vi "SE Initialization VI.vi"(8 "error in (no error)":errorcluster, 10 "Custom XML":string, 11 "Device Item Ref in":T1 format="%.0x") -> (0 "error out":errorcluster, 3 "Device Item Ref out":T1 format="%.0x")   [LabVIEW 2018, in "Chassis TimeSync System Explorer.lvlib"]
uses:
  Chassis TimeSync System Explorer.lvlib
  <vilib>/NI Veristand/Custom Device API/Custom Device Item Ref.ctl
  <vilib>/NI Veristand/Custom Device API/Custom Device Channel Type.ctl
  Shared/Constants.vi
  <vilib>/NI Veristand/Custom Device API/Custom Device API.lvlib
  Shared/Chassis TimeSync Shared.lvlib
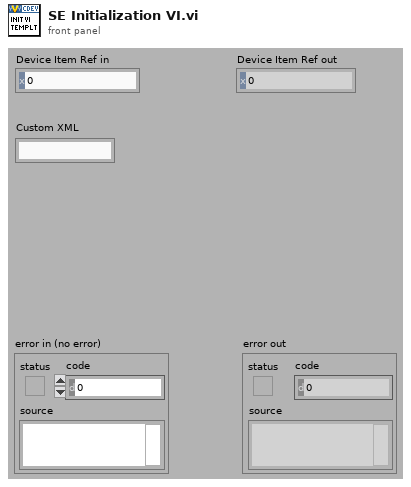
[diagram p1: front panel]
types:
  T1 = typedef "Custom Device API.lvlib/Custom Device Item Ref.ctl" = u64
  T2 = typedef "Custom Device API.lvlib/Custom Device Channel Type.ctl" = enum16{"Input", "Output"}
  T3 = typedef "Chassis TimeSync Shared.lvlib/Channel.ctl" = cluster{"Name":string, "Units":string, "Default":dbl, "Description":string}
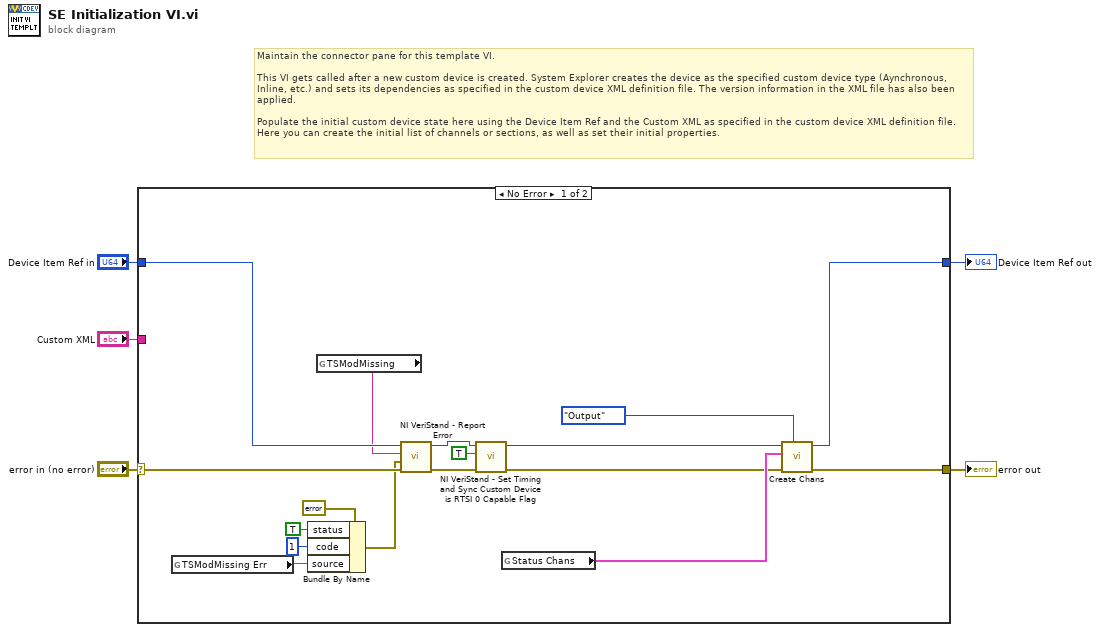
[diagram p0: block diagram]
diagram:
  # "Maintain the connector pane for this template VI.\n\nThis VI gets called after a new custom device is created. System Explorer creates the device as the specified custom device type (Aynchronous, Inline, etc.) and sets its dependencies as specified in the custom device XML definition file. The version information in the XML file has also been applied.\n\nPopulate the initial custom device state here using the Device Item Ref and the Custom XML as specified in the custom device XML definition file. Here you can create the initial list of channels or sections, as well as set their initial properties."
  n1 = case shown="No Error" "error in (no error)" {
    selector: "error in (no error)" -> [w18 w24]
    tunnel: [w11 w24] -> w5
    tunnel: [w10 w23] -> w3
    tunnel: "Device Item Ref in" -> [w20 w23]
    tunnel: "Custom XML" -> [_ _]
    frame No Error {
      n2 = global read "Constants.vi" "TSModMissing Err"() -> (w13:string)
      n3 = Bundle By Name(cluster=errorcluster {"status"=FALSE, "code"=0, "source"=""} ("error constant"), "status"=TRUE, "code"=1, "source"=w13) -> (w12:errorcluster)
      n4 = global read "Constants.vi" "TSModMissing"() -> (w17:string)
      n5 = call <vilib>:"NI VeriStand - Report Error.vi"("error in (no error)"=w18, "New Error"=w12, "Error ID"=w17, "Node Ref in"=w20) -> ("error out"=w21:errorcluster, "Node Ref out"=w19:T1)  [unwired: 6 in]
      n6 = call <vilib>:"NI VeriStand - Set Timing and Sync Custom Device is RTSI 0 Capable Flag.vi"("error in (no error)"=w21, "Is RTSI 0 Capable"=TRUE, "Device Ref in"=w19) -> ("error out"=w6:errorcluster, "Device Ref out"=w7:T1)  [unwired: 7 in]
      n7 = global read "Constants.vi" "Status Chans"() -> (w9:T3[])
      n8 = call "Create Chans.vi"("Type"=Custom_Device_Channel_Type."Output", "error in (no error)"=w6, "Channels"=w9, "Section Ptr"=w7) -> ("error out"=w11:errorcluster, "Section Ptr dup"=w10:T1)  [unwired: 6 in]
    }
    frame Error {
    }
  }
  "error out" <- w5
  "Device Item Ref out" <- w3
